vi "TB-Update History.vi"(0 "history in":cluster{"time":dbl[], "value":dbl[]}[](array[cluster]), 5 "history values":dbl[](array[numeric]), 7 "Index":i32, 9 "Time":dbl) -> (4 "history out":cluster{dbl[], dbl[]}[](array[cluster]))   [LabVIEW 2020]
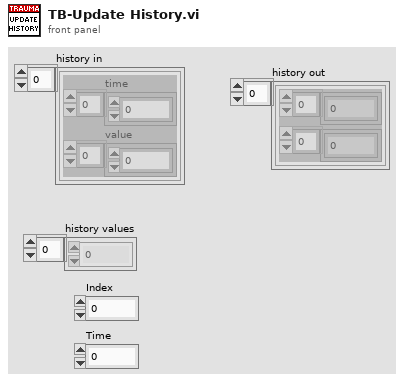
[diagram p1: front panel]
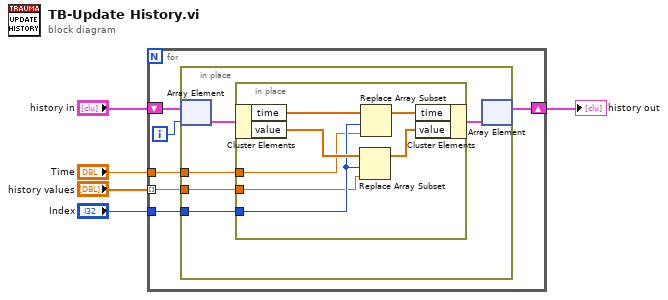
[diagram p0: block diagram]
diagram:
  n1 = for {
    shift-right: [w9] -> w4
    shift-left: "history in" -> [w11]
    tunnel: "history values" -> [w6] mode=indexing
    tunnel: "Index" -> [w8]
    tunnel: "Time" -> [w7]
    i -> [w10]
    n2 = in-place {
      in-place-border: w8 -> [w14]
      in-place-border: w7 -> [w13]
      in-place-border: w6 -> [w12]
      n3 = in-place-array #1(w11, w10) -> (w16:cluster{"time":dbl[], "value":dbl[]})
      n4 = in-place {
        in-place-border: w14 -> [w19]
        in-place-border: w13 -> [w18]
        in-place-border: w12 -> [w17]
        n5 = in-place-cluster #2(w16) -> ("time"=w23:dbl[], "value"=w21:dbl[])
        n6 = Replace Array Subset(array=w21, new element=w17, index=w19) -> (w20:dbl[])
        n7 = Replace Array Subset(array=w23, new element=w18, index=w19) -> (w22:dbl[])
        n8 = in-place-cluster #2("time"=w22, "value"=w20) -> (w15:cluster{"time":dbl[], "value":dbl[]})
      }
      n9 = in-place-array #1(w15) -> (w9:cluster{"time":dbl[], "value":dbl[]}[])  [unwired: 1 out]
    }
  }
  "history out" <- w4
